vi "ImageClose.vi"(8 "error in (no error)":errorcluster, 11 "Image in":refnum<class "Image.lvclass">) -> (0 "error out":errorcluster, 3 "Image out":refnum<class "Image.lvclass">)   [LabVIEW 2012, in "Image.lvclass"]
uses:
  classes/Image.lvclass
  classes/Image.lvclass/Image.ctl
panel:
  out "Numeric":i32
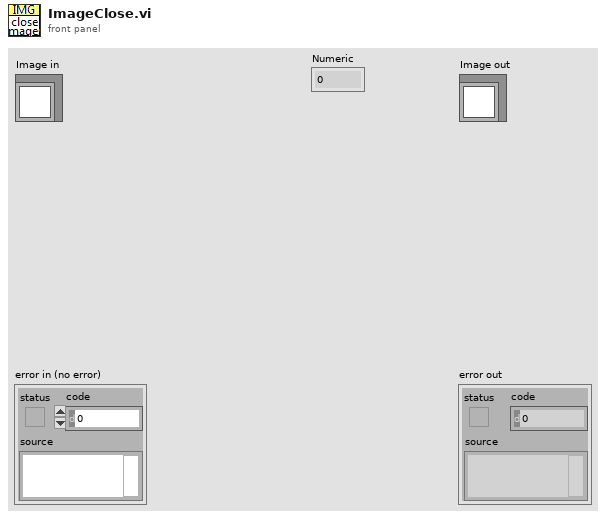
[diagram p1: front panel]
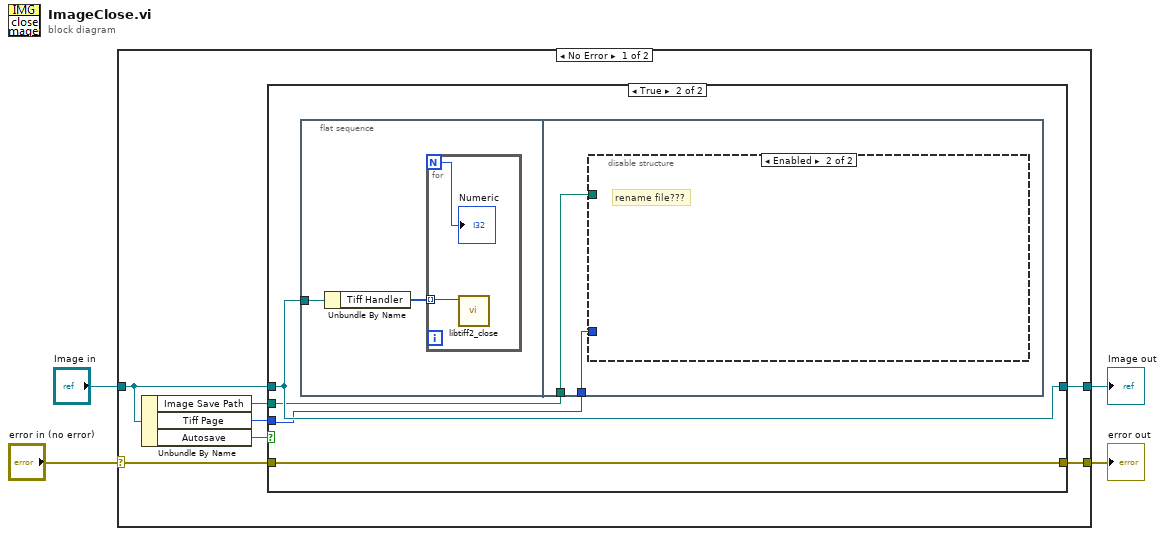
[diagram p0: block diagram]
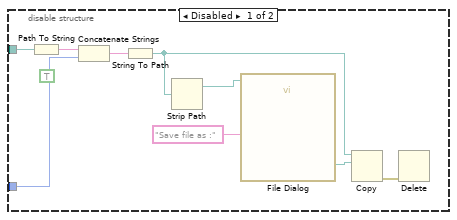
[diagram p3: hidden frame]
diagram:
  n1 = case shown="No Error" "error in (no error)" {
    selector: "error in (no error)" -> [w11 w34]
    tunnel: [w10 w34] -> w3
    tunnel: [w7 w33] -> w2
    tunnel: "Image in" -> [w8 w33]
    frame No Error {
      n2 = Unbundle By Name(w8) -> ("Image Save Path"=w6:path, "Tiff Page"=w5:u32, "Autosave"=w9:bool)
      n3 = case shown="True" w9 {
        tunnel: w11 -> [w12 w16]
        tunnel: [w12 w16] -> w10
        tunnel: w8 -> [w13 w17]
        tunnel: [w13 w17] -> w7
        tunnel: w6 -> [_ w15]
        tunnel: w5 -> [_ w14]
        frame False {
        }
        frame True {
          n4 = flat-sequence {
            tunnel: w17 -> [w18]
            tunnel: w15 -> [w23]
            tunnel: w14 -> [w22]
            frame #0 {
              n5 = Unbundle By Name(w18) -> ("Tiff Handler"=w19:u32[])
              n6 = for {
                N -> [w20]
                tunnel: w19 -> [w21] mode=indexing
                n7 = call "libtiff2_close.vi"("Handle"=w21) -> ()  [unwired: 9 in, 1 out]
                "Numeric" <- w20
              }
            }
            frame #1 {
              n8 = disable-structure shown="Enabled" {
                disable-tunnel: w23 -> [w26 _]
                disable-tunnel: w22 -> [w25 _]
                frame Disabled {
                  (unwired) TRUE ("overwrite (F)")
                  n9 = Path To String(path=w26) -> (string=w28:string)
                  n10 = Concatenate Strings(w28, w25) -> (w29:string)
                  n11 = String To Path(string=w29) -> (path=w30:path)
                  n12 = Strip Path(path=w30) -> (stripped path=w31:path)  [unwired: 1 out]
                  n13 = call "File Dialog"("start path"=w31, "prompt"="Save file as :") -> ("selected path"=w32:path)  [unwired: 10 in, 3 out]
                  n14 = Copy(10:w32, 11:w30) -> (0:w27:errorcluster)  [unwired: 3 in, 2 out]
                  n15 = Delete(error in=w27) -> ()  [unwired: 4 in, 3 out]
                }
                frame Enabled {
                  # "rename file???"
                }
              }
            }
          }
        }
      }
    }
    frame Error {
    }
  }
  "error out" <- w3
  "Image out" <- w2
